vi "Test C.vi"(1 "board image":T1) -> (0 "pass?":T2)   [LabVIEW 2018]
doc: "Test a GPIB board image."
uses:
  Common/Pass Fail Boolean.ctl
  Common/Board Image.ctl
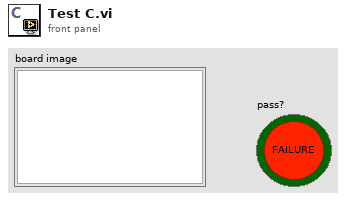
[diagram p1: front panel]
types:
  T1 = typedef "Board Image.ctl" = picture
  T2 = typedef "Pass Fail Boolean.ctl" = bool
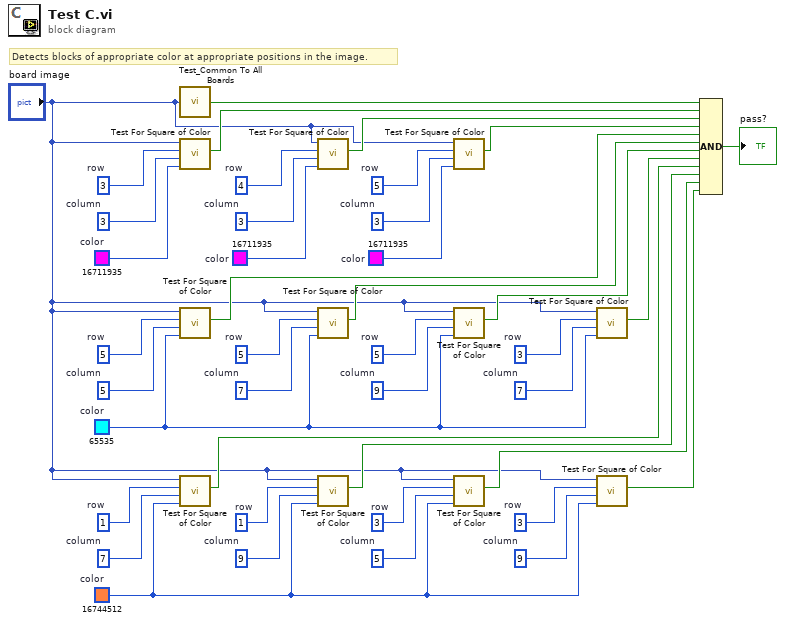
[diagram p0: block diagram]
diagram:
  w4 = i16 9  # column
  w5 = i16 3  # row
  w9 = i16 7  # column
  w8 = i16 3  # row
  w16 = i16 5  # column
  w15 = i16 3  # row
  w17 = i16 9  # column
  w18 = i16 1  # row
  w20 = i16 7  # column
  w19 = i16 1  # row
  w3 = u32 16744512  # color
  w30 = i16 9  # column
  w31 = i16 5  # row
  w29 = i16 7  # column
  w28 = i16 5  # row
  w26 = i16 5  # column
  w27 = i16 5  # row
  w7 = u32 65535  # color
  w33 = i16 3  # column
  w32 = i16 5  # row
  w34 = u32 16711935  # color
  w36 = i16 3  # column
  w37 = i16 4  # row
  w35 = u32 16711935  # color
  w40 = i16 3  # column
  w39 = i16 3  # row
  w41 = u32 16711935  # color
  # "Detects blocks of appropriate color at appropriate positions in the image."
  n1 = call "Test_Common To All Boards.vi"("board image"="board image") -> ("pass?"=w13:T2)
  n2 = call "Test For Square of Color.vi"("color"=w41, "column"=w40, "row"=w39, "board image"="board image") -> ("pass?"=w38:T2)  [unwired: 7 in]
  n3 = call "Test For Square of Color.vi"("color"=w7, "column"=w26, "row"=w27, "board image"="board image") -> ("pass?"=w23:T2)  [unwired: 7 in]
  n4 = call "Test For Square of Color.vi"("color"=w3, "column"=w20, "row"=w19, "board image"="board image") -> ("pass?"=w10:T2)  [unwired: 7 in]
  n5 = call "Test For Square of Color.vi"("color"=w35, "column"=w36, "row"=w37, "board image"="board image") -> ("pass?"=w25:T2)  [unwired: 7 in]
  n6 = call "Test For Square of Color.vi"("color"=w7, "column"=w29, "row"=w28, "board image"="board image") -> ("pass?"=w22:T2)  [unwired: 7 in]
  n7 = call "Test For Square of Color.vi"("color"=w3, "column"=w17, "row"=w18, "board image"="board image") -> ("pass?"=w11:T2)  [unwired: 7 in]
  n8 = call "Test For Square of Color.vi"("color"=w34, "column"=w33, "row"=w32, "board image"="board image") -> ("pass?"=w24:T2)  [unwired: 7 in]
  n9 = call "Test For Square of Color.vi"("color"=w7, "column"=w30, "row"=w31, "board image"="board image") -> ("pass?"=w21:T2)  [unwired: 7 in]
  n10 = call "Test For Square of Color.vi"("color"=w3, "column"=w16, "row"=w15, "board image"="board image") -> ("pass?"=w12:T2)  [unwired: 7 in]
  n11 = call "Test For Square of Color.vi"("color"=w7, "column"=w9, "row"=w8, "board image"="board image") -> ("pass?"=w6:T2)  [unwired: 7 in]
  n12 = call "Test For Square of Color.vi"("color"=w3, "column"=w4, "row"=w5, "board image"="board image") -> ("pass?"=w1:T2)  [unwired: 7 in]
  n13 = Compound Arithmetic op=AND(w13, w38, w25, w24, w23, w22, w21, w6, w10, w11, w12, w1) -> (→"pass?":T2)
